vi "Display Export In Tree.vi"(0 "Build Analyzer in":refnum<class "Build Analyzer.lvclass">, 5 "Tree":refnum<vi>, 7 "Product Name":string, 11 "error in (no error)":errorcluster) -> (4 "Build Analyzer out":refnum<class "Build Analyzer.lvclass">, 15 "error out":errorcluster)   [LabVIEW 2017, in "CL_G3_VIComponentBuilder.lvlib" / "Build Analyzer.lvclass"]
doc: "Displays the hierarchy of compoenents to be built in a tree structure."
uses:
  Build Analyzer.lvclass
  Build Analyzer.lvclass/Build Analyzer.ctl
  Accessors/Read Product Name - Unique Name.vi
  <userlib>/_Cirrus Logic/LabVIEW Container/Source/Container/Get Child.vi
  <userlib>/_Cirrus Logic/LabVIEW Container/Source/Container/Container.lvclass
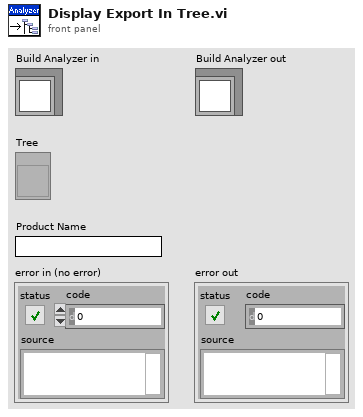
[diagram p1: front panel]
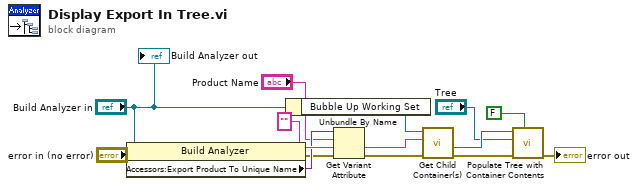
[diagram p0: block diagram]
diagram:
  n1 = property class="Build Analyzer"(reference="Build Analyzer in", error in="error in (no error)") -> (error out=w5:errorcluster, "Accessors:Export Product To Unique Name"=w8:variant)  [unwired: 1 out]
  n2 = Unbundle By Name("Build Analyzer in") -> ("Bubble Up Working Set"=w11:refnum<data-value>)
  n3 = Get Variant Attribute(Variant=w8, name="Product Name", default value (empty Variant)="" ("element"), error in=w5) -> (value=w7:string, error out=w4:errorcluster)  [unwired: 2 out]
  n4 = call-poly <userlib>:"Get Child Container(s).vi"("error in (no error)"=w4, "Container Name"=w7, "Container"=w11) -> ("error out"=w3:errorcluster, "Child Container"=w13:refnum<data-value>)  [unwired: 5 in, 2 out]
  n5 = call <userlib>:"Populate Tree with Container Contents.vi"("Open all Children? (T)"=FALSE, "error in (no error)"=w3, "Tree"="Tree", "Container Reference"=w13) -> ("error out"=→"error out":errorcluster)  [unwired: 6 in, 1 out]
  "Build Analyzer out" <- "Build Analyzer in"
